vi "Get Paragraphs.Text.vi"(8 "error in (no error)":errorcluster, 11 "xwpfHeader in":refnum<class "xwpfHeader_Footer.lvclass">) -> (0 "error out":errorcluster, 2 "Paragraphs.Text":string, 3 "xwpfHeader out":refnum<class "xwpfHeader_Footer.lvclass">)   [LabVIEW 2017, in "Word_Specific.lvlib" / "xwpfHeader_Footer.lvclass"]
uses:
  xwpfHeader_Footer.lvclass
  xwpfHeader_Footer.lvclass/xwpfHeader_Footer.ctl
  xwpfParagraph/Get Runs.Text.vi
  xwpfParagraph/xwpfParagraph.lvclass
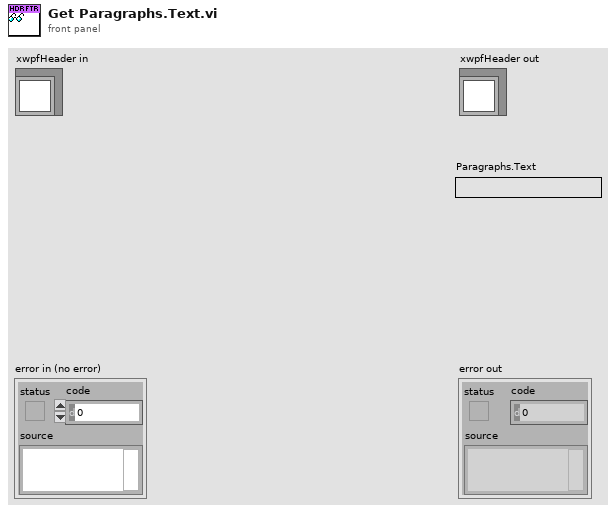
[diagram p1: front panel]
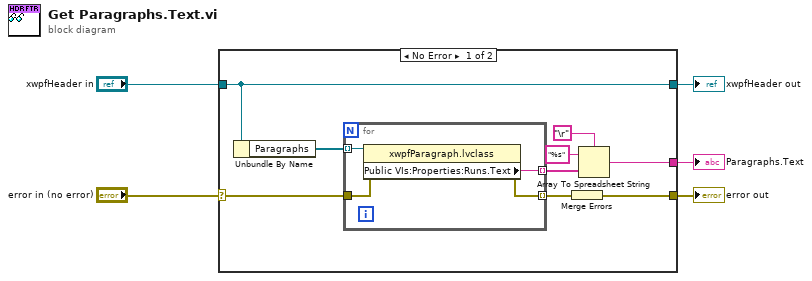
[diagram p0: block diagram]
diagram:
  n1 = case shown="No Error" "error in (no error)" {
    selector: "error in (no error)" -> [w8 w19]
    tunnel: [w6 w19] -> w4
    tunnel: [w14 w20] -> w2
    tunnel: "xwpfHeader in" -> [w14 w20]
    tunnel: [w7 _] -> w1
    frame No Error {
      n2 = Unbundle By Name(w14) -> ("Paragraphs"=w13:refnum<class "xwpfParagraph.lvclass">[])
      n3 = for {
        tunnel: w13 -> [w18] mode=indexing
        tunnel: [w17] -> w10 mode=indexing
        tunnel: [w16] -> w9 mode=indexing
        tunnel: w8 -> [w15]
        n4 = property class="xwpfParagraph.lvclass"(reference=w18, error in=w15) -> (error out=w16:errorcluster, "Public VIs:Properties:Runs.Text"=w17:string)  [unwired: 1 out]
      }
      n5 = Merge Errors(w9) -> (w6:errorcluster)
      n6 = Array To Spreadsheet String(delimiter (Tab)="\r", array=w10, 3:"%s" ("format string")) -> (spreadsheet string=w7:string)
    }
    frame Error {
    }
  }
  "error out" <- w4
  "xwpfHeader out" <- w2
  "Paragraphs.Text" <- w1
